vi "Send Last Stop Event.vi"(8 "error in (no error)":errorcluster, 11 "Actor in":refnum<class "Actor.lvclass">) -> (0 "error out":errorcluster, 3 "Actor  out":refnum<class "Actor.lvclass">)   [LabVIEW 2014, in "Observable Actor.lvlib" / "Observable Actor.lvclass"]
uses:
  Observable Actor.lvclass
  <vilib>/ActorFramework/Actor/Actor.lvclass
  Observable Actor.lvclass/Observable Actor.ctl
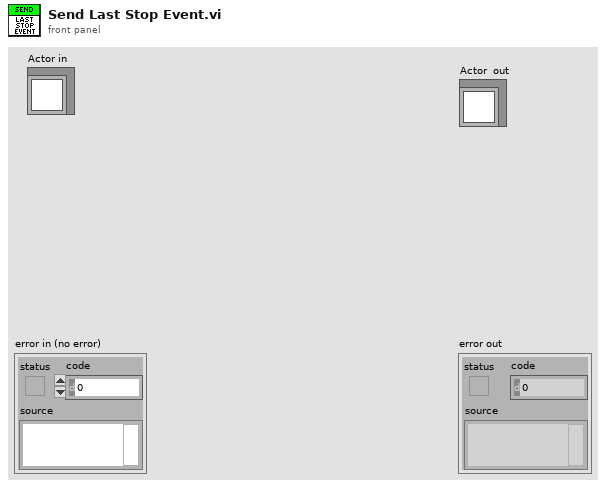
[diagram p1: front panel]
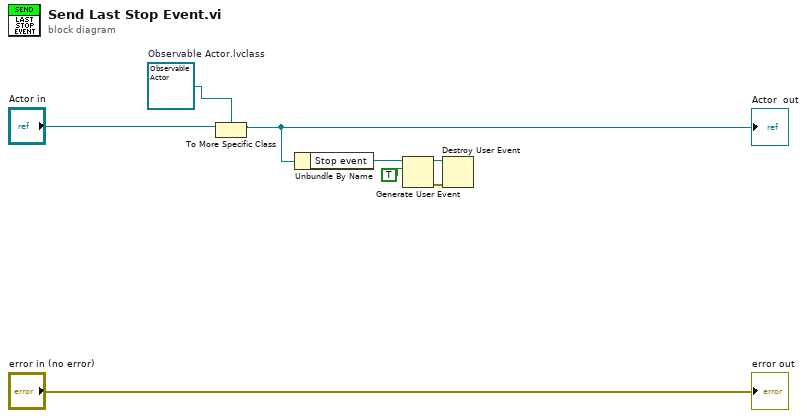
[diagram p0: block diagram]
diagram:
  w1 = refnum<class "Observable Actor.lvclass"> refnum  # Observable Actor.lvclass
  n1 = To More Specific Class(target class=w1, reference="Actor in") -> (specific class reference=w8:refnum<class "Observable Actor.lvclass">)  [unwired: 1 in, 1 out]
  "Actor  out" <- w8
  n2 = Unbundle By Name(w8) -> ("Stop event"=w6:refnum<user-event>)
  n3 = Generate User Event(user event=w6, event data cluster=TRUE ("event data")) -> (user event out=w4:refnum<user-event>, error out=w3:errorcluster)  [unwired: 2 in]
  n4 = Destroy User Event(user event=w4, error in=w3) -> ()  [unwired: 1 out]
  "error out" <- "error in (no error)"
